vi "Read Meta Data (UDP Clst).vi"(6 "options":T4={"ignore timeout error"=TRUE, "timeout ms (1000)"=1000, "max size (548)"=548}, 8 "error in":errorcluster, 11 "connection info in":T2) -> (0 "error out":errorcluster, 1 "meta data":T1[](array[typedef]), 3 "connection info out":T2, 4 "data info":T3)   [LabVIEW 2010, in "NI STM.lvlib"]
doc: "This VI reads the meta data information from a remote computer. Use this VI to retrieve the variable names and types that a remote computer exports.\n\nThis VI parses the data and returns a cluster containing the meta data information.\n\nCopyright 2015, 2016, 2017 National Instruments Corporation\n\nLicensed under the Apache License, Version 2.0 (the \"License\"); you may not use this file except in compliance with the License.\n\n You may obtain a copy of the License at\n\n http://www.apache.org/licenses/LICENSE-2.0\n\nUnless required by applicable law or agreed to in writing, software distributed under the License is distributed on an \"AS IS\" BASIS, WITHOUT WARRANTIES OR CONDITIONS OF ANY KIND, either express or implied.\n\nSee the License for the specific language governing permissions and limitations under the License."
uses:
  NI STM.lvlib
  UDP Read Options.ctl
  UDP Data Info.ctl
  UDP Connection Info.ctl
  SubVIs/MetaDataElement.ctl
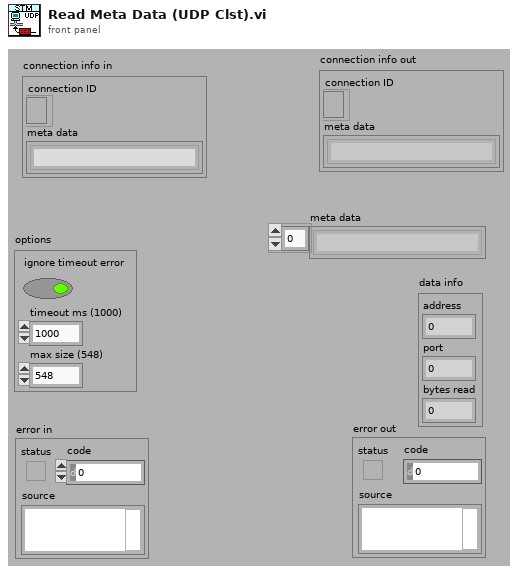
[diagram p1: front panel]
types:
  T1 = typedef "NI STM.lvlib/MetaDataElement.ctl" = string
  T2 = typedef "NI STM.lvlib/UDP Connection Info.ctl" = cluster{"connection ID":refnum<k16>, "meta data":T1[]}
  T3 = typedef "NI STM.lvlib/UDP Data Info.ctl" = cluster{"address":u32, "port":u16, "bytes read":i32}
  T4 = typedef "NI STM.lvlib/UDP Read Options.ctl" = cluster{"ignore timeout error":bool, "timeout ms (1000)":i32, "max size (548)":i32}
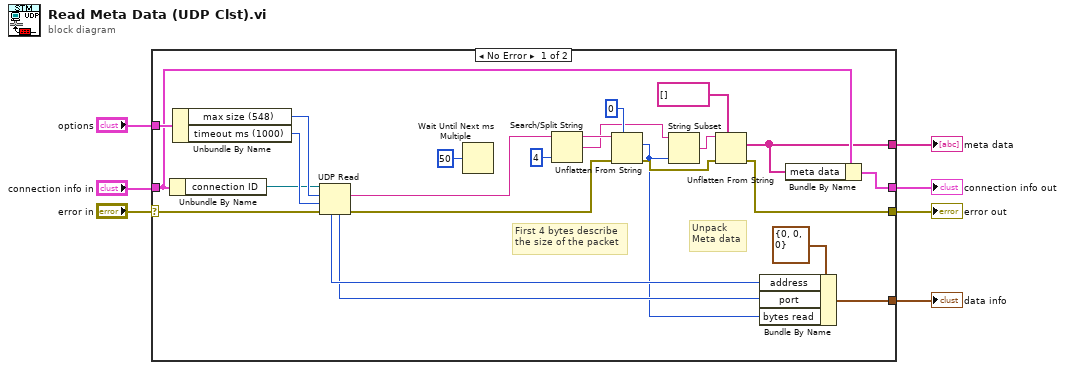
[diagram p0: block diagram]
diagram:
  n1 = case shown="No Error" "error in" {
    selector: "error in" -> [w30 w32]
    tunnel: [w14 _] -> w2
    tunnel: [w31 w32] -> w7
    tunnel: "connection info in" -> [w16 w33]
    tunnel: [w17 w33] -> w3
    tunnel: "options" -> [w18 _]
    tunnel: [w8 _] -> w1
    frame No Error {
      # "First 4 bytes describe\nthe size of the packet"
      # "Unpack\nMeta data"
      n2 = Unbundle By Name(w16) -> ("connection ID"=w19:refnum<k16>)
      n3 = Unbundle By Name(w18) -> ("max size (548)"=w21:i32, "timeout ms (1000)"=w20:i32)
      n4 = UDP Read(connection ID=w19, max size (548)=w21, timeout ms (25000)=w20, 8:w30) -> (data out=w29:string, error out=w22:errorcluster, 4:w10:u16, 6:w11:u32)  [unwired: 1 out]
      n5 = Wait Until Next ms Multiple(millisecond multiple=u32 50) -> ()  [unwired: 1 out]
      n6 = Search/Split String(string=w29, offset (0)=4) -> (substring before match=w27:string, match + rest of string=w24:string)  [unwired: 2 out]
      n7 = Unflatten From String(type=0, binary string=w27, error in (no error)=w22) -> (value=w9:i32, error out=w13:errorcluster)  [unwired: 3 out]
      n8 = String Subset(string=w24, length (rest)=w9) -> (substring=w25:string)  [unwired: 1 out]
      n9 = Unflatten From String(type=T1[] [] ("Meta data"), binary string=w25, error in (no error)=w13) -> (value=w14:T1[], error out=w31:errorcluster)  [unwired: 3 out]
      n10 = Bundle By Name(cluster=T3 {"address"=0, "port"=0, "bytes read"=0} ("Data Info"), "address"=w11, "port"=w10, "bytes read"=w9) -> (w8:T3)
      n11 = Bundle By Name(cluster=w16, "meta data"=w14) -> (w17:T2)
    }
    frame Error {
    }
  }
  "error out" <- w7
  "data info" <- w1
  "connection info out" <- w3
  "meta data" <- w2
